vi "MainLogLoop.vi"(8 "error in (no error)":errorcluster, 10 "Sensors":T10={"Gyro"={"DevStatus"={"status"=FALSE, "code"=0, "source"=""}, "Analog Channel"=enum."Invalid", "Offset"=0.0, "Gain (VoltsPerDegree/Second)"=0.0, "Gyro Type"=enum."Analog", "Handle"=0, "SPI Bus"=enum."Invalid", "Device Found"=FALSE, "Sample Rate"=1.0, "Calibrate On Open"=FALSE}, "Encoders"={"Left Drive CAN"={"DeviceStatus"={"status"=FALSE, "code"=0, "source"=""}, "Type"=enum."PWM", "PWM"={"PWM Channel"=enum."PWM 1", "DeadBand"={"Name"="", "maxPositivePwm"=0, "minPositivePwm"=0, "centerPwm"=0, "maxNegativePwm"=0, "minNegativePwm"=0, "angularRange"=0}}, "CAN"={"Device Number"=0, "Control Mode"=enum."Percent VBus", "Semaphore"=refnum, "Max Vout"=12.0, "TalonSRX Control Mode"=enum."Percent VBus"}, "Invert"=FALSE}, "Right Drive CAN"={"DeviceStatus"={"status"=FALSE, "code"=0, "source"=""}, "Type"=enum."PWM", "PWM"={"PWM Channel"=enum."PWM 1", "DeadBand"={"Name"="", "maxPositivePwm"=0, "minPositivePwm"=0, "centerPwm"=0, "maxNegativePwm"=0, "minNegativePwm"=0, "angularRange"=0}}, "CAN"={"Device Number"=0, "Control Mode"=enum."Percent VBus", "Semaphore"=refnum, "Max Vout"=12.0, "TalonSRX Control Mode"=enum."Percent VBus"}, "Invert"=FALSE}, "Strafe CAN"={"DeviceStatus"={"status"=FALSE, "code"=0, "source"=""}, "Type"=enum."PWM", "PWM"={"PWM Channel"=enum."PWM 1", "DeadBand"={"Name"="", "maxPositivePwm"=0, "minPositivePwm"=0, "centerPwm"=0, "maxNegativePwm"=0, "minNegativePwm"=0, "angularRange"=0}}, "CAN"={"Device Number"=0, "Control Mode"=enum."Percent VBus", "Semaphore"=refnum, "Max Vout"=12.0, "TalonSRX Control Mode"=enum."Percent VBus"}, "Invert"=FALSE}, "Elevator CAN"={"DeviceStatus"={"status"=FALSE, "code"=0, "source"=""}, "Type"=enum."PWM", "PWM"={"PWM Channel"=enum."PWM 1", "DeadBand"={"Name"="", "maxPositivePwm"=0, "minPositivePwm"=0, "centerPwm"=0, "maxNegativePwm"=0, "minNegativePwm"=0, "angularRange"=0}}, "CAN"={"Device Number"=0, "Control Mode"=enum."Percent VBus", "Semaphore"=refnum, "Max Vout"=12.0, "TalonSRX Control Mode"=enum."Percent VBus"}, "Invert"=FALSE}}, "Switches"={"Elevator Top"={"DevStatus"={"status"=FALSE, "code"=0, "source"=""}, "DIO Channel"=enum."DIO 1", "CntIndex"=enum."Invalid", "Normally Closed"=FALSE}, "Elevator Bottom"={"DevStatus"={"status"=FALSE, "code"=0, "source"=""}, "DIO Channel"=enum."DIO 1", "CntIndex"=enum."Invalid", "Normally Closed"=FALSE}, "Claw Outside"={"DevStatus"={"status"=FALSE, "code"=0, "source"=""}, "DIO Channel"=enum."DIO 1", "CntIndex"=enum."Invalid", "Normally Closed"=FALSE}, "Tote Touch"={"DevStatus"={"status"=FALSE, "code"=0, "source"=""}, "DIO Channel"=enum."DIO 1", "CntIndex"=enum."Invalid", "Normally Closed"=FALSE}}, "Arm Capper Pot"={"DevStatus"={"status"=FALSE, "code"=0, "source"=""}, "Analog Channel"=enum."Invalid", "Invert Output"=FALSE}, "Arm Angle Pot"={"DevStatus"={"status"=FALSE, "code"=0, "source"=""}, "Analog Channel"=enum."Invalid", "Invert Output"=FALSE}, "Sonar"={"Front"={"AIDeviceRef"={"DevStatus"={"status"=FALSE, "code"=0, "source"=""}, "Analog Channel"=enum."Invalid"}, "Scaling factor (V/in)"=0.0098, "Average Bits"=3}, "Back"={"AIDeviceRef"={"DevStatus"={"status"=FALSE, "code"=0, "source"=""}, "Analog Channel"=enum."Invalid"}, "Scaling factor (V/in)"=0.0098, "Average Bits"=3}}} {"Sonar"."Back"."Average Bits" max=15; "Sonar"."Front"."Average Bits" max=15; "Gyro"."Sample Rate" min=0.25 max=100.0 step=0.25}, 11 "Actuators":T1={"Drive"={"DevStatus"={"status"=FALSE, "code"=0, "source"=""}, "Motors[]"=[], "Square Inputs"=FALSE, "Max Output"=1.0}, "Strafe"={"DeviceStatus"={"status"=FALSE, "code"=0, "source"=""}, "Type"=enum."PWM", "PWM"={"PWM Channel"=enum."Invalid", "DeadBand"={"Name"="", "maxPositivePwm"=0, "minPositivePwm"=0, "centerPwm"=0, "maxNegativePwm"=0, "minNegativePwm"=0, "angularRange"=0}}, "CAN"={"Device Number"=0, "Control Mode"=enum."Percent VBus", "Semaphore"=refnum, "Max Vout"=12.0, "TalonSRX Control Mode"=enum."Percent VBus"}, "Invert"=FALSE}, "Elevator Left"={"DeviceStatus"={"status"=FALSE, "code"=0, "source"=""}, "Type"=enum."PWM", "PWM"={"PWM Channel"=enum."Invalid", "DeadBand"={"Name"="", "maxPositivePwm"=0, "minPositivePwm"=0, "centerPwm"=0, "maxNegativePwm"=0, "minNegativePwm"=0, "angularRange"=0}}, "CAN"={"Device Number"=0, "Control Mode"=enum."Percent VBus", "Semaphore"=refnum, "Max Vout"=12.0, "TalonSRX Control Mode"=enum."Percent VBus"}, "Invert"=FALSE}, "Elevator Right"={"DeviceStatus"={"status"=FALSE, "code"=0, "source"=""}, "Type"=enum."PWM", "PWM"={"PWM Channel"=enum."Invalid", "DeadBand"={"Name"="", "maxPositivePwm"=0, "minPositivePwm"=0, "centerPwm"=0, "maxNegativePwm"=0, "minNegativePwm"=0, "angularRange"=0}}, "CAN"={"Device Number"=0, "Control Mode"=enum."Percent VBus", "Semaphore"=refnum, "Max Vout"=12.0, "TalonSRX Control Mode"=enum."Percent VBus"}, "Invert"=FALSE}, "Arm Clapper"={"DeviceStatus"={"status"=FALSE, "code"=0, "source"=""}, "Type"=enum."PWM", "PWM"={"PWM Channel"=enum."Invalid", "DeadBand"={"Name"="", "maxPositivePwm"=0, "minPositivePwm"=0, "centerPwm"=0, "maxNegativePwm"=0, "minNegativePwm"=0, "angularRange"=0}}, "CAN"={"Device Number"=0, "Control Mode"=enum."Percent VBus", "Semaphore"=refnum, "Max Vout"=12.0, "TalonSRX Control Mode"=enum."Percent VBus"}, "Invert"=FALSE}, "Arm Angle"={"DeviceStatus"={"status"=FALSE, "code"=0, "source"=""}, "Type"=enum."PWM", "PWM"={"PWM Channel"=enum."Invalid", "DeadBand"={"Name"="", "maxPositivePwm"=0, "minPositivePwm"=0, "centerPwm"=0, "maxNegativePwm"=0, "minNegativePwm"=0, "angularRange"=0}}, "CAN"={"Device Number"=0, "Control Mode"=enum."Percent VBus", "Semaphore"=refnum, "Max Vout"=12.0, "TalonSRX Control Mode"=enum."Percent VBus"}, "Invert"=FALSE}, "Arm Roller Left"={"DeviceStatus"={"status"=FALSE, "code"=0, "source"=""}, "Type"=enum."PWM", "PWM"={"PWM Channel"=enum."Invalid", "DeadBand"={"Name"="", "maxPositivePwm"=0, "minPositivePwm"=0, "centerPwm"=0, "maxNegativePwm"=0, "minNegativePwm"=0, "angularRange"=0}}, "CAN"={"Device Number"=0, "Control Mode"=enum."Percent VBus", "Semaphore"=refnum, "Max Vout"=12.0, "TalonSRX Control Mode"=enum."Percent VBus"}, "Invert"=FALSE}, "Arm Roller Right"={"DeviceStatus"={"status"=FALSE, "code"=0, "source"=""}, "Type"=enum."PWM", "PWM"={"PWM Channel"=enum."Invalid", "DeadBand"={"Name"="", "maxPositivePwm"=0, "minPositivePwm"=0, "centerPwm"=0, "maxNegativePwm"=0, "minNegativePwm"=0, "angularRange"=0}}, "CAN"={"Device Number"=0, "Control Mode"=enum."Percent VBus", "Semaphore"=refnum, "Max Vout"=12.0, "TalonSRX Control Mode"=enum."Percent VBus"}, "Invert"=FALSE}, "Wiper"={"DeviceStatus"={"status"=FALSE, "code"=0, "source"=""}, "Type"=enum."PWM", "PWM"={"PWM Channel"=enum."Invalid", "DeadBand"={"Name"="", "maxPositivePwm"=0, "minPositivePwm"=0, "centerPwm"=0, "maxNegativePwm"=0, "minNegativePwm"=0, "angularRange"=0}}, "CAN"={"Device Number"=0, "Control Mode"=enum."Percent VBus", "Semaphore"=refnum, "Max Vout"=12.0, "TalonSRX Control Mode"=enum."Percent VBus"}, "Invert"=FALSE}}) -> (0 "error out":errorcluster)   [LabVIEW 2015]
uses:
  Main/Robot Global Data.vi
  Utilities/Sensor Refname.ctl
  packet types.ctl
  Utilities/Sensor Refname to String.vi
  <vilib>/Rock Robotics/SystemInterfaces/AI/FPGA_AIChannel.ctl
  <vilib>/Rock Robotics/WPI/Gyro/WPI_GyroDevRef.ctl
  <vilib>/Rock Robotics/WPI/CAN/Jaguar/SubVIs/WPI_CANJaguar_ControlMode.ctl
  <vilib>/Rock Robotics/WPI/CAN/TalonSRX/WPI_CANTalonSRX_APIControlMode.ctl
  <vilib>/Rock Robotics/SystemInterfaces/DIO/FPGA_DIOPWMChannel.ctl
  <vilib>/Rock Robotics/WPI/PWM/WPI_PWMDeadband.ctl
  <vilib>/Rock Robotics/WPI/MotorControl/WPI_MotorControlType.ctl
  <vilib>/Rock Robotics/WPI/MotorControl/WPI_MotorControlDeviceRef.ctl
  <vilib>/Rock Robotics/SystemInterfaces/DIO/FPGA_DIOChannel.ctl
  <vilib>/Rock Robotics/SystemInterfaces/Counter/FPGA_CounterCtrSystemIndex.ctl
  <vilib>/Rock Robotics/WPI/Switch/WPI_SwitchDevRef.ctl
  <vilib>/Rock Robotics/WPI/Potentiometer/WPI_PotentiometerDevRef.ctl
  <vilib>/Rock Robotics/WPI/AnalogChannel/WPI_AnalogChannelDevRef.ctl
  <vilib>/Rock Robotics/WPI/Ultrasonic/WPI_SonarMB1010AnalogDeviceRef.ctl
  Utilities/Sensors.ctl
  <vilib>/Rock Robotics/WPI/RobotDrive/WPI_RobotDriveDevRef.ctl
  Utilities/Actuators.ctl
  <vilib>/Rock Robotics/SystemInterfaces/spilib/spi_bus.ctl
panel:
  out "result string to log":string
  # "Testing outputs:"
  # "Analog"
  # "XRS"
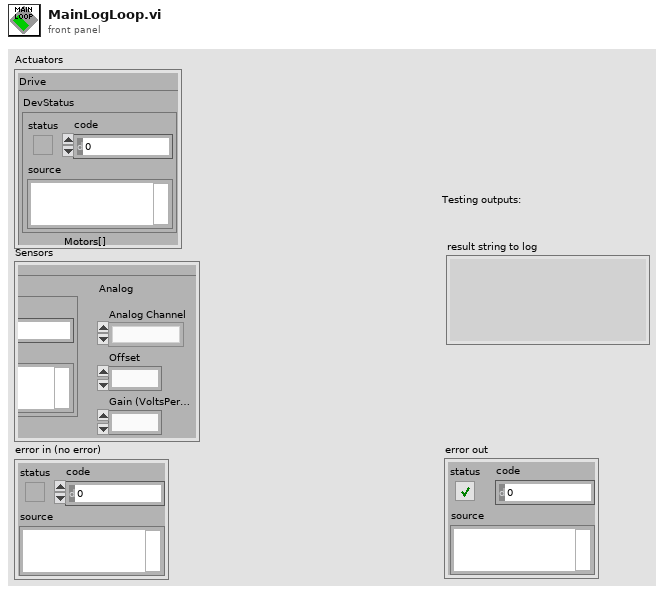
[diagram p1: front panel]
types:
  T1 = typedef "Actuators.ctl" = cluster{"Drive":T2, "Strafe":T3, "Elevator Left":T3, "Elevator Right":T3, "Arm Clapper":T3, "Arm Angle":T3, "Arm Roller Left":T3, "Arm Roller Right":T3, "Wiper":T3}
  T2 = typedef "WPI_RobotDriveDevRef.ctl" = cluster{"DevStatus":errorcluster, "Motors[]":T3[], "Square Inputs":bool, "Max Output":dbl}
  T3 = typedef "WPI_MotorControlDeviceRef.ctl" = cluster{"DeviceStatus":errorcluster, "Type":T4, "PWM":cluster{"PWM Channel":T5, "DeadBand":T6}, "CAN":cluster{"Device Number":u8, "Control Mode":T7, "Semaphore":T8, "Max Vout":dbl, "TalonSRX Control Mode":T9}, "Invert":bool}
  T4 = typedef "WPI_MotorControlType.ctl" = enum16{"PWM", "CAN", "CANTalonSRX"}
  T5 = typedef "FPGA_DIOPWMChannel.ctl" = enum8{"PWM 0", "PWM 1", "PWM 2", "PWM 3", "PWM 4", "PWM 5", "PWM 6", "PWM 7", "PWM 8", "PWM 9", "PWM MXP 0", "PWM MXP 1", "PWM MXP 2", "PWM MXP 3", "PWM MXP 4", "PWM MXP 5", "PWM MXP 6", "PWM MXP 7", "PWM MXP 8", "PWM MXP 9", "Invalid"}
  T6 = typedef "WPI_PWMDeadband.ctl" = cluster{"Name":string, "maxPositivePwm":i32, "minPositivePwm":i32, "centerPwm":i32, "maxNegativePwm":i32, "minNegativePwm":i32, "angularRange":u16}
  T7 = typedef "WPI_CANJaguar_ControlMode.ctl" = enum8{"Percent VBus", "Current", "Speed", "Position", "Voltage"}
  T8 = typedef "Semaphore RefNum" = refnum<k1>
  T9 = typedef "WPI_CANTalonSRX_APIControlMode.ctl" = enum8{"Percent VBus", "Speed", "Position", "Slave", "Unchanged / Invalid", "Voltage Compensation", "Current", "Motion Profile"}
  T10 = typedef "Sensors.ctl" = cluster{"Gyro":T11, "Encoders":cluster{"Left Drive CAN":T3, "Right Drive CAN":T3, "Strafe CAN":T3, "Elevator CAN":T3}, "Switches":cluster{"Elevator Top":T14, "Elevator Bottom":T14, "Claw Outside":T14, "Tote Touch":T14}, "Arm Capper Pot":T17, "Arm Angle Pot":T17, "Sonar":cluster{"Front":T18, "Back":T18}}
  T11 = typedef "WPI_GyroDevRef.ctl" = cluster{"DevStatus":errorcluster, "Analog Channel":T12, "Offset":dbl, "Gain (VoltsPerDegree/Second)":dbl, "Gyro Type":enum16{"Analog", "XRS450"}, "Handle":i32, "SPI Bus":T13, "Device Found":bool, "Sample Rate":dbl, "Calibrate On Open":bool}
  T12 = typedef "FPGA_AIChannel.ctl" = enum8{"AI 0", "AI 1", "AI 2", "AI 3", "AI MXP 0", "AI MXP 1", "AI MXP 2", "AI MXP 3", "Invalid"}
  T13 = typedef "spi_bus.ctl" = enum16{"SPI On-Board, CS0", "SPI On-Board, CS1", "SPI On-Board, CS2", "SPI On-Board, CS3", "SPI MXP", "Invalid"}
  T14 = typedef "WPI_SwitchDevRef.ctl" = cluster{"DevStatus":errorcluster, "DIO Channel":T15, "CntIndex":T16, "Normally Closed":bool}
  T15 = typedef "FPGA_DIOChannel.ctl" = enum8{"DIO 0", "DIO 1", "DIO 2", "DIO 3", "DIO 4", "DIO 5", "DIO 6", "DIO 7", "DIO 8", "DIO 9", "DIO MXP 0", "DIO MXP 1", "DIO MXP 2", "DIO MXP 3", "DIO MXP 4", "DIO MXP 5", "DIO MXP 6", "DIO MXP 7", "DIO MXP 8", "DIO MXP 9", "DIO MXP 10", "DIO MXP 11", "DIO MXP 12", "DIO MXP 13", "DIO MXP 14", "DIO MXP 15", "Invalid"}
  T16 = typedef "FPGA_CounterCtrSystemIndex.ctl" = enum8{"Ctr 0", "Ctr 1", "Ctr 2", "Ctr 3", "Ctr 4", "Ctr 5", "Ctr 6", "Ctr 7", "Invalid"}
  T17 = typedef "WPI_PotentiometerDevRef.ctl" = cluster{"DevStatus":errorcluster, "Analog Channel":T12, "Invert Output":bool}
  T18 = typedef "WPI_SonarMB1010AnalogDeviceRef.ctl" = cluster{"AIDeviceRef":T19, "Scaling factor (V/in)":dbl, "Average Bits":u8}
  T19 = typedef "WPI_AnalogChannelDevRef.ctl" = cluster{"DevStatus":errorcluster, "Analog Channel":T12}
  T20 = typedef "packet types.ctl" = enum16{"Log line", "Open File", "Send Header", "Set Time", "Send to LCD"}
  T21 = typedef "Sensor Refname.ctl" = enum16{"Gyro", "Elevator Top LS", "Elevator Bottom LS", "Claw Outside LS", "Left Drive Encoder", "Right Drive Encoder", "Strafe Encoder", "Elevator Encoder", "Ultrasonic Forward", "Ultrasonic Back", "Arm Angle POT", "Arm Clapper POT", "Accelerometer", "Tote LS", "DIP 1", "DIP 2", "DIP 3", "DIP 4"}
  T22 = typedef "WPI_SerialPortRef.ctl" = cluster{"DevStatus":errorcluster, "Serial Port Name":refnum<visa-resource-name>}
  T23 = cluster{"Left Drive CAN":T3, "Right Drive CAN":T3, "Strafe CAN":T3, "Elevator CAN":T3}
  T24 = typedef "WPI_AccelerometerDevRef.ctl" = cluster{"DevStatus":errorcluster, "Scaling":T25, "Analog Channels":T26, "I2C Bus":T27, "SPI Bus":T13, "Accel Range":T28, "ADXL Axes":T29, "Handle":i32, "Device Address":u8, "Accel Type":enum16{"Analog", "ADXL345 I2C", "ADXL345 SPI", "Internal", "ADXL362 SPI"}}
  T25 = typedef "WPI_AccelerometerScaling.ctl" = cluster{"Gain (VoltsPerG)":dbl, "Center Voltage":dbl}
  T26 = typedef "WPI_AccelerometerAnalogChannels.ctl" = cluster{"X-Axis":T12, "Y-Axis":T12, "Z-Axis":T12}
  T27 = typedef "i2c_bus.ctl" = enum16{"I2C On-Board", "I2C MXP", "Invalid"}
  T28 = typedef "ADXL345 Range.ctl" = u8
  T29 = typedef "WPI_AccelerometerADXL345 Axes.ctl" = cluster{"X-Axis":bool, "Y-Axis":bool, "Z-Axis":bool}
  T30 = typedef "WPI_DriverStationRobotMode2.ctl" = enum16{"Autonomous Disabled", "Autonomous Enabled", "Teleop Disabled", "Teleop Enabled", "Disconnected", "Finish", "Test Disabled", "Test Enabled", "Emergency Stopped"}
  T31 = cluster{"X-Axis":dbl, "Y-Axis":dbl, "Z-Axis":dbl}
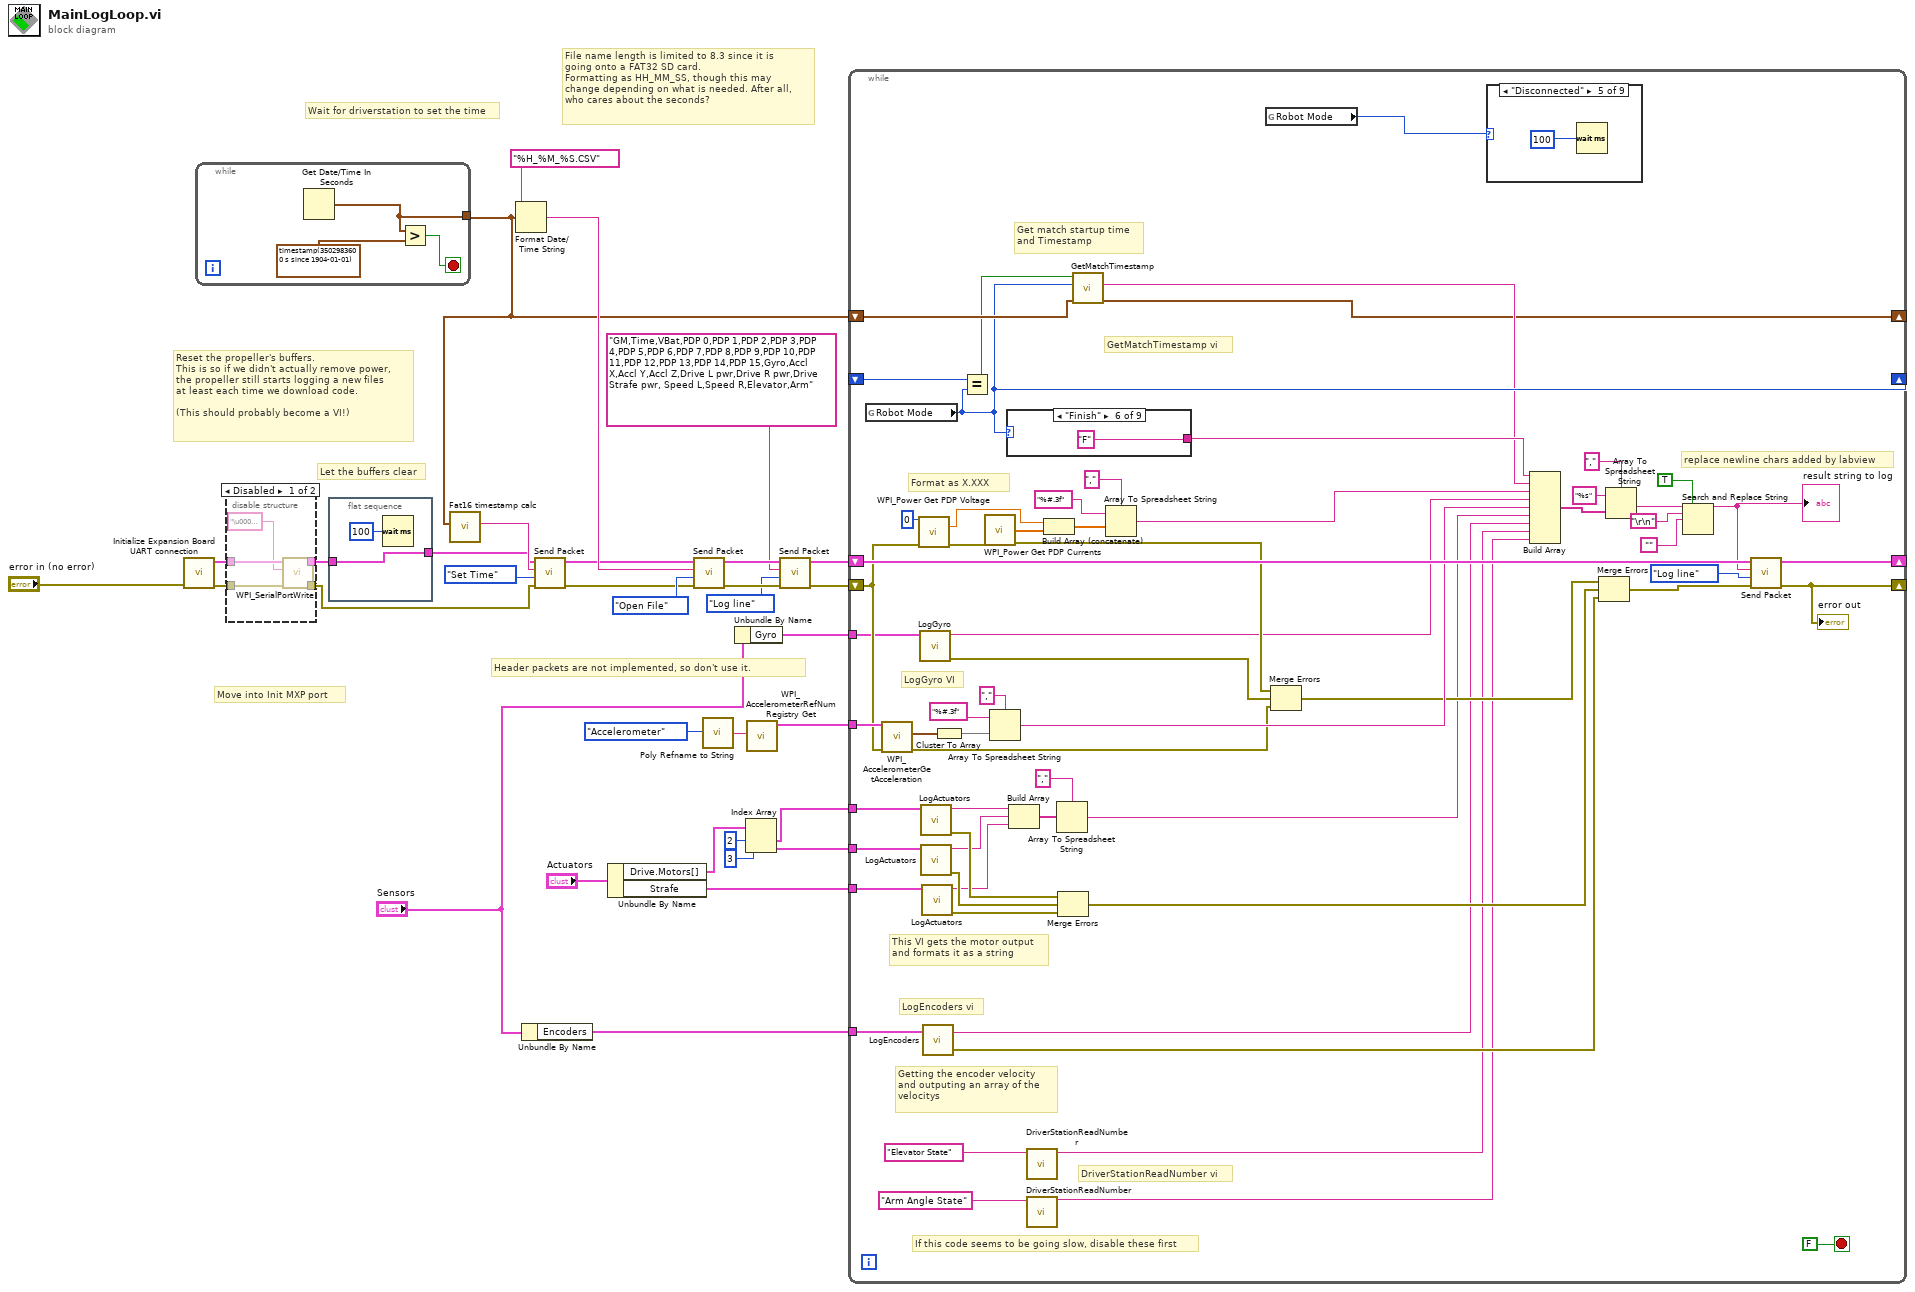
[diagram p0: block diagram]
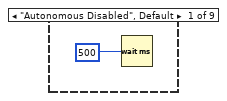
[diagram p3: hidden frame]
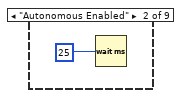
[diagram p4: hidden frame]
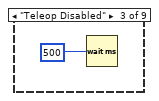
[diagram p5: hidden frame]
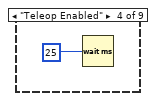
[diagram p6: hidden frame]
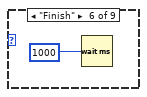
[diagram p7: hidden frame]
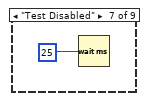
[diagram p8: hidden frame]
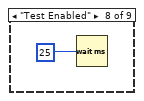
[diagram p9: hidden frame]
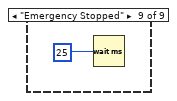
[diagram p10: hidden frame]
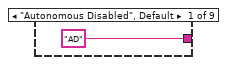
[diagram p11: hidden frame]
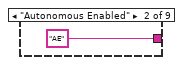
[diagram p12: hidden frame]
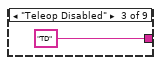
[diagram p13: hidden frame]
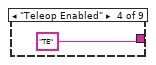
[diagram p14: hidden frame]
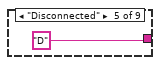
[diagram p15: hidden frame]
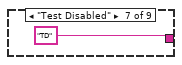
[diagram p16: hidden frame]
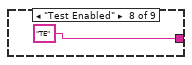
[diagram p17: hidden frame]
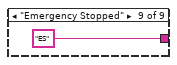
[diagram p18: hidden frame]
diagram:
  # "Move into Init MXP port"
  # "Let the buffers clear"
  # "Reset the propeller's buffers.\nThis is so if we didn't actually remove power,\nthe propeller still starts logging a new files \nat least each time we download code.\n\n(This should probably become a VI!)"
  # "File name length is limited to 8.3 since it is \ngoing onto a FAT32 SD card. \nFormatting as HH_MM_SS, though this may\nchange depending on what is needed. After all,\nwho cares about the seconds?"
  # "Wait for driverstation to set the time"
  # "Header packets are not implemented, so don't use it."
  n1 = call "Initialize Expansion Board UART connection.vi"("error in (no error)"="error in (no error)") -> ("error out"=w6:errorcluster, "SerialPortRef"=w5:T22)  [unwired: 9 in]
  n2 = while {
    tunnel: [w34] -> w8
    stop <- w35 stop-if-true
    n3 = Get Date/Time In Seconds() -> (seconds since 1Jan1904=w34:timestamp)
    n4 = Greater?(x=w34, y=timestamp(3502983600 s since 1904-01-01)) -> (0:w35:bool)
  }
  n5 = disable-structure shown="Disabled" {
    disable-tunnel: w6 -> [w41 w42]
    disable-tunnel: w5 -> [w40 w43]
    disable-tunnel: [w38 w43] -> w3
    disable-tunnel: [w37 w42] -> w2
    frame Disabled {
      n6 = call <vilib>:"WPI_SerialPortWrite.vi"("error in (no error)"=w41, "Buffer"="\u0004\u0004", "SerialPortRef"=w40) -> ("error out"=w37:errorcluster, "SerialPortRef"=w38:T22)  [unwired: 6 in, 1 out]
    }
    frame Enabled {
    }
  }
  n7 = flat-sequence {
    tunnel: [w45] -> w4
    tunnel: w3 -> [w45]
    frame #0 {
      n8 = Wait (ms)(milliseconds to wait=u32 100) -> ()  [unwired: 1 out]
    }
  }
  n9 = call "Fat16 timestamp calc.vi"("time stamp"=w8) -> ("timestamp as string"=w9:string)  [unwired: 10 in]
  n10 = Format Date/Time String(time format string (%c)="%H_%M_%S.CSV", seconds (now)=w8) -> (date/time string=w15:string)  [unwired: 1 in]
  n11 = Unbundle By Name("Sensors") -> ("Encoders"=w1:T23)
  n12 = call "Send Packet.vi"("error in (no error)"=w2, 7:packet_types."Set Time", "Log string"=w9, "SerialPortRef"=w4) -> ("error out"=w11:errorcluster, "SerialPortRef out"=w10:T22)  [unwired: 4 in]
  n13 = Unbundle By Name("Actuators") -> ("Drive.Motors[]"=w20:T3[], "Strafe"=w21:T3)
  n14 = call "Send Packet.vi"("error in (no error)"=w11, 7:packet_types."Open File", "Log string"=w15, "SerialPortRef"=w10) -> ("error out"=w31:errorcluster, "SerialPortRef out"=w32:T22)  [unwired: 4 in]
  n15 = call-poly "Poly Refname to String.vi"("Sensor Refnames"=Sensor_Refname."Accelerometer" ("Sensor Refname")) -> ("Refname"=w27:string)
  n16 = Unbundle By Name("Sensors") -> ("Gyro"=w19:T11)
  n17 = Index Array(array=w20, index #1=2 ("index"), index #2=3 ("index")) -> (element #1=w25:T3, element #2=w24:T3)
  n18 = call <vilib>:"WPI_AccelerometerRefNum Registry Get.vi"("refnum name"=w27) -> ("AccelerometerDevRef"=w28:T24)  [unwired: 9 in, 1 out]
  n19 = call "Send Packet.vi"("error in (no error)"=w31, 7:packet_types."Log line", "Log string"="GM,Time,VBat,PDP 0,PDP 1,PDP 2,PDP 3,PDP 4,PDP 5,PDP 6,PDP 7,PDP 8,PDP 9,PDP 10,PDP 11,PDP 12,PDP 13,PDP 14,PDP 15,Gyro,Accl X,Accl Y,Accl Z,Drive L pwr,Drive R pwr,Drive Strafe pwr, Speed L,Speed R,Elevator,Arm", "SerialPortRef"=w32) -> ("error out"=w26:errorcluster, "SerialPortRef out"=w29:T22)  [unwired: 4 in]
  n20 = while {
    shift-right: [w80] -> _
    shift-left: w26 -> [w92]
    shift-right: [w107] -> _
    shift-left: w29 -> [w108]
    tunnel: w28 -> [w104]
    tunnel: w21 -> [w62]
    tunnel: w19 -> [w73]
    tunnel: w25 -> [w64]
    tunnel: w24 -> [w63]
    shift-right: [w68] -> _
    shift-left: _ -> [w103]
    shift-right: [w65] -> _
    shift-left: w8 -> [w69]
    tunnel: w1 -> [w70]
    stop <- FALSE stop-if-true
    # "DriverStationReadNumber vi"
    # "This VI gets the motor output\nand formats it as a string"
    # "GetMatchTimestamp vi"
    # "Get match startup time \nand Timestamp"
    # "LogEncoders vi"
    # "Getting the encoder velocity\nand outputing an array of the \nvelocitys"
    # "LogGyro VI"
    # "If this code seems to be going slow, disable these first"
    # "replace newline chars added by labview"
    # "Format as X.XXX"
    n21 = global read "Robot Global Data.vi" "Robot Mode"() -> (w68:T30)
    n22 = call <vilib>:"WPI_AccelerometerGetAcceleration.vi"("error in"=w92, "AccelerometerDevRef"=w104) -> ("error out"=w74:errorcluster, "Accelerations"=w76:T31)  [unwired: 7 in, 1 out]
    n23 = call <vilib>:"WPI_Power Get PDP Voltage.vi"("Power Distribution Panel (0)"=u8 0, "error in"=w92) -> ("voltage (V)"=w100:dbl, "error out"=w93:errorcluster)  [unwired: 12 in]
    n24 = call "LogGyro.vi"("GyroDevRef"=w73) -> ("error out"=w71:errorcluster, "Gyro Angle"=w72:string)  [unwired: 9 in]
    n25 = call "LogActuators.vi"("MotorControlDevRef"=w64) -> ("error out"=w60:errorcluster, "resulting string"=w55:string)  [unwired: 9 in]
    n26 = call "LogActuators.vi"("MotorControlDevRef"=w63) -> ("error out"=w59:errorcluster, "resulting string"=w56:string)  [unwired: 9 in]
    n27 = call "LogActuators.vi"("MotorControlDevRef"=w62) -> ("error out"=w58:errorcluster, "resulting string"=w57:string)  [unwired: 9 in]
    n28 = call "LogEncoders.vi"("input cluster"=w70) -> ("error out"=w50:errorcluster, "concatenated string"=w51:string)  [unwired: 9 in]
    n29 = Cluster To Array(cluster=w76) -> (array=w75:dbl[])
    n30 = Equal?(x=w103, y=w68) -> (x = y?=w67:bool)
    n31 = call <vilib>:"WPI_Power Get PDP Currents.vi"("error in"=w93) -> ("all currents (A)"=w91:dbl[], "error out"=w89:errorcluster)  [unwired: 12 in, 1 out]
    n32 = Array To Spreadsheet String(delimiter (Tab)=",", array=w75, 3:"%#.3f" ("format string")) -> (spreadsheet string=w94:string)
    n33 = case shown="\"Finish\"" w68 {
      tunnel: ["AD" "AE" "TD" "TE" "D" "F" "TD" "TE" "ES"] -> w90
      frame "Autonomous Disabled", Default {
      }
      frame "Autonomous Enabled" {
      }
      frame "Teleop Disabled" {
      }
      frame "Teleop Enabled" {
      }
      frame "Disconnected" {
      }
      frame "Finish" {
      }
      frame "Test Disabled" {
      }
      frame "Test Enabled" {
      }
      frame "Emergency Stopped" {
      }
    }
    n34 = Build Array(w55, w56, w57) -> (w54:string[])
    n35 = call "DriverStationReadNumber.vi"("Name"="Elevator State") -> ("output string"=w48:string)  [unwired: 10 in]
    n36 = call "DriverStationReadNumber.vi"("Name"="Arm Angle State") -> ("output string"=w46:string)  [unwired: 10 in]
    n37 = Build Array (concatenate)(w100, w91) -> (w99:dbl[])
    n38 = Array To Spreadsheet String(delimiter (Tab)=",", array=w54) -> (spreadsheet string=w52:string)  [unwired: 1 in]
    n39 = Merge Errors(w60, w59, w58) -> (w61:errorcluster)
    n40 = call "GetMatchTimestamp.vi"("seconds since 1Jan1904"=w69, "Robot Mode"=w68, "Boolean"=w67) -> ("seconds since 1Jan1904 2"=w65:timestamp, "Match Timestamp"=w66:string)  [unwired: 7 in]
    n41 = Array To Spreadsheet String(delimiter (Tab)=",", array=w99, 3:"%#.3f" ("format string")) -> (spreadsheet string=w95:string)
    n42 = global read "Robot Global Data.vi" "Robot Mode"() -> (w87:T30)
    n43 = Merge Errors(w89, w71, w74) -> (w79:errorcluster)
    n44 = case shown="\"Disconnected\"" w87 {
      frame "Autonomous Disabled", Default {
        n45 = Wait (ms)(milliseconds to wait=u32 500) -> ()  [unwired: 1 out]
      }
      frame "Autonomous Enabled" {
        n46 = Wait (ms)(milliseconds to wait=u32 25) -> ()  [unwired: 1 out]
      }
      frame "Teleop Disabled" {
        n47 = Wait (ms)(milliseconds to wait=u32 500) -> ()  [unwired: 1 out]
      }
      frame "Teleop Enabled" {
        n48 = Wait (ms)(milliseconds to wait=u32 25) -> ()  [unwired: 1 out]
      }
      frame "Disconnected" {
        n49 = Wait (ms)(milliseconds to wait=u32 100) -> ()  [unwired: 1 out]
      }
      frame "Finish" {
        n50 = Wait (ms)(milliseconds to wait=u32 1000) -> ()  [unwired: 1 out]
      }
      frame "Test Disabled" {
        n51 = Wait (ms)(milliseconds to wait=u32 25) -> ()  [unwired: 1 out]
      }
      frame "Test Enabled" {
        n52 = Wait (ms)(milliseconds to wait=u32 25) -> ()  [unwired: 1 out]
      }
      frame "Emergency Stopped" {
        n53 = Wait (ms)(milliseconds to wait=u32 25) -> ()  [unwired: 1 out]
      }
    }
    n54 = Build Array(w90, w66, w95, w72, w94, w52, w51, w48, w46) -> (w96:string[])
    n55 = Merge Errors(w79, w61, w50) -> (w86:errorcluster)
    n56 = Array To Spreadsheet String(delimiter (Tab)=",", array=w96, 3:"%s" ("format string")) -> (spreadsheet string=w82:string)
    n57 = Search and Replace String(replace all?=TRUE ("replace all? (F)"), input string=w82, search string="\r\n", replace string="") -> (result string=w81:string)  [unwired: 4 in, 3 out]
    "result string to log" <- w81
    n58 = call "Send Packet.vi"("error in (no error)"=w86, 7:packet_types."Log line", "Log string"=w81, "SerialPortRef"=w108) -> ("error out"=w80:errorcluster, "SerialPortRef out"=w107:T22)  [unwired: 4 in]
    "error out" <- w80
  }
